vi "Read Refs.vi"(11 "Project Stuff in":refnum<class "Project Stuff.lvclass">) -> (2 "Refs":T1)   [LabVIEW 2020, in "_Shared.lvlib" / "Project Stuff.lvclass"]
uses:
  Project Stuff.lvclass
  Refs.ctl
  VI.ctl
  Library.ctl
  Project Stuff.lvclass/Project Stuff.ctl
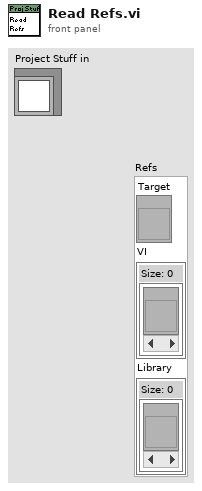
[diagram p1: front panel]
types:
  T1 = typedef "_Shared.lvlib/Project Stuff.lvclass/Refs.ctl" = cluster{"Target":refnum<vi>, "VI":T2, "Library":T3}
  T2 = typedef "_Shared.lvlib/Project Stuff.lvclass/VI.ctl" = set{refnum<vi>}
  T3 = typedef "_Shared.lvlib/Project Stuff.lvclass/Library.ctl" = set{refnum<vi>}
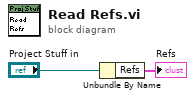
[diagram p0: block diagram]
diagram:
  n1 = Unbundle By Name("Project Stuff in") -> ("Refs"=→"Refs":T1)
